vi "validate configuration.vi"(8 "error in":errorcluster, 11 "engine configuration in":refnum<class "engine configuration.lvclass">) -> (0 "error out":errorcluster, 3 "engine configuration out":refnum<class "engine configuration.lvclass">)   [LabVIEW 2013, in "engine configuration.lvclass"]
doc: "This VI returns an error if the configuration object is in a state that is incompatible with execution."
uses:
  engine configuration.lvclass
  <vilib>/NI/Tag Bus Module Framework/root configuration/TBM configuration.lvclass
  engine configuration.lvclass/engine configuration.ctl
  <vilib>/NI/CEF/CEF_TreeControl/NISE_CEF_TreeControl.lvlib
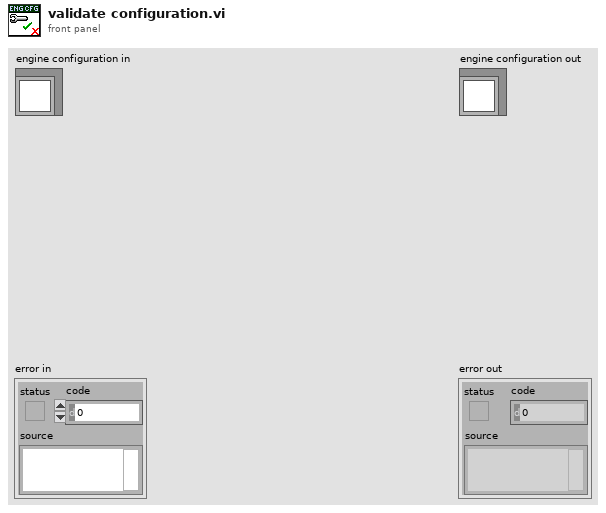
[diagram p1: front panel]
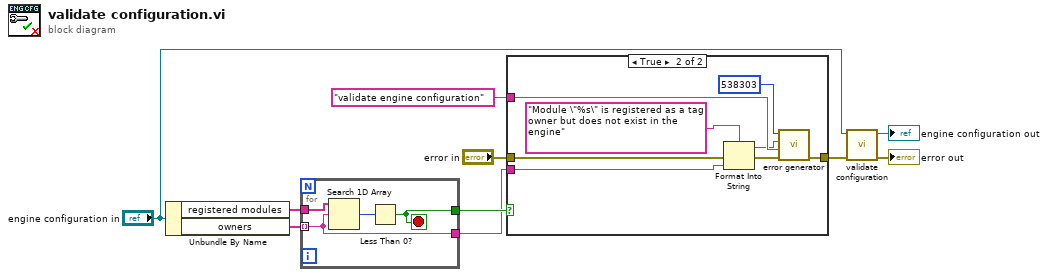
[diagram p0: block diagram]
diagram:
  n1 = Unbundle By Name("engine configuration in") -> ("registered modules"=w4:string[], "owners"=w7:string[])
  n2 = for {
    tunnel: w7 -> [w11] mode=indexing
    tunnel: w4 -> [w14]
    tunnel: [w12] -> w6
    tunnel: [w11] -> w2
    stop <- w12 stop-if-true
    n3 = Search 1D Array(1D array=w14, element=w11) -> (index of element=w13:i32)  [unwired: 1 in]
    n4 = Less Than 0?(x=w13) -> (x < 0?=w12:bool)
  }
  n5 = case shown="True" w6 {
    tunnel: "error in" -> [w15 w20]
    tunnel: [w15 w23] -> w5
    tunnel: "validate engine configuration" ("source") -> [_ w21]
    tunnel: w2 -> [_ w17]
    frame False {
    }
    frame True {
      n6 = Format Into String(format string="Module \"%s\" is registered as a tag owner but does not exist in the engine", error in=w20, w17) -> (resulting string=w18:string, error out=w19:errorcluster)  [unwired: 1 in]
      n7 = call <vilib>:"error generator.vi"("error in"=w19, "source"=w21, "append error message"=w18, "error code (0)"=538303) -> ("error out"=w23:errorcluster)  [unwired: 5 in]
    }
  }
  n8 = call-parent "validate configuration.vi"("error in"=w5, "configuration in"="engine configuration in") -> ("error out"=→"error out":errorcluster, "configuration out"=→"engine configuration out":refnum<class "engine configuration.lvclass">)  [unwired: 8 in]
